vi "Read.vi"(8 "error in (no error)":errorcluster, 11 "Serial in":refnum<class "Serial.lvclass">) -> (0 "error out":errorcluster, 2 "Output":string, 3 "Serial out":refnum<class "Serial.lvclass">)   [LabVIEW 2019, in "Serial.lvclass"]
uses:
  Serial.lvclass
  Serial.lvclass/Serial.ctl
  d80e3772-2fb9-4f29-8b62-39276b340b93.vi
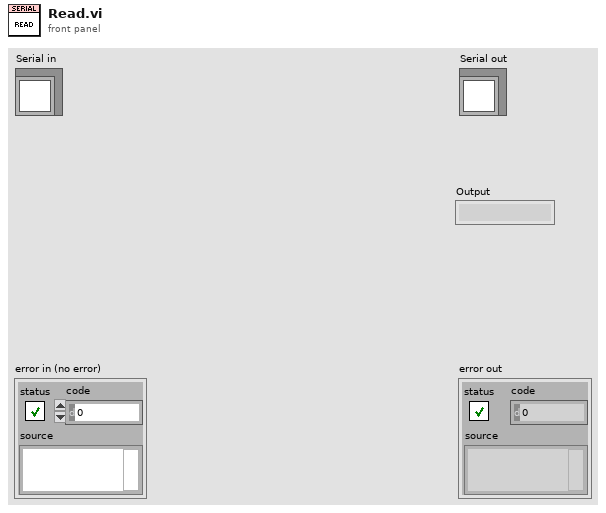
[diagram p1: front panel]
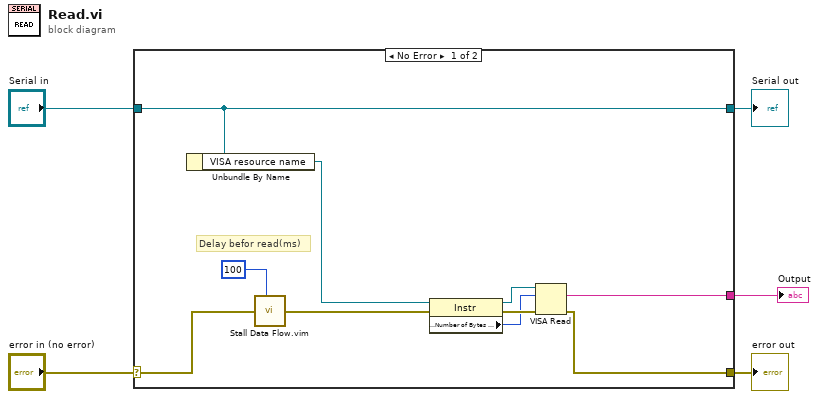
[diagram p0: block diagram]
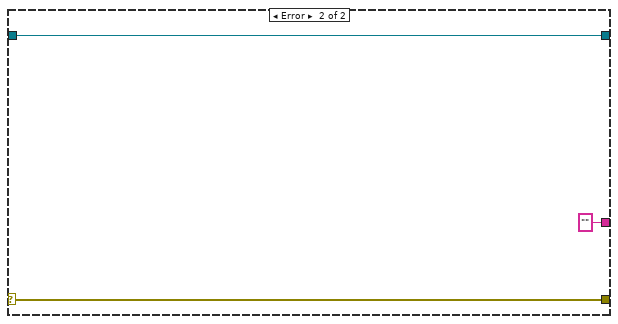
[diagram p2: hidden frame]
diagram:
  n1 = case shown="No Error" "error in (no error)" {
    selector: "error in (no error)" -> [w8 w18]
    tunnel: [w7 w18] -> w4
    tunnel: [w10 w17] -> w2
    tunnel: "Serial in" -> [w10 w17]
    tunnel: [w6 "" ("read buffer")] -> w1
    frame No Error {
      # "Delay befor read(ms)"
      n2 = Unbundle By Name(w10) -> ("VISA resource name"=w9:refnum<visa-resource-name>)
      n3 = call "Stall Data Flow.vim"("value in"=w8, "milliseconds to wait"=u32 100) -> ("value out"=w15:errorcluster)  [unwired: 1 out]
      n4 = property class="Instr"(reference=w9, error in=w15) -> (reference out=w13:refnum<visa-resource-name>, error out=w14:errorcluster, "Serial Settings:Number of Bytes at Serial Port"=w12:u32)
      n5 = VISA Read(VISA resource name=w13, byte count=w12, error in (no error)=w14) -> (read buffer=w6:string, error out=w7:errorcluster)  [unwired: 2 out]
    }
    frame Error {
    }
  }
  "error out" <- w4
  "Serial out" <- w2
  "Output" <- w1
